vi "OpenDISession.vi"(8 "error in (no error)":errorcluster, 10 "gRPCid":T5, 11 "DIOSessions In":T1={"Array of DI Sessions"=[], "Array of DO Sessions"=[], "Stream ReadDI"={"gRPCid ReadDI"=0, "DISessionName"="", "Stream Status ReadDI"=FALSE, "Async Stop ReadDI Queue"=refnum, "DI Task"="", "ms to wait"=500}}) -> (0 "error out":errorcluster, 3 "DIOSessions Out":T1={"Array of DI Sessions"=[], "Array of DO Sessions"=[], "Stream ReadDI"={"gRPCid ReadDI"=0, "DISessionName"="", "Stream Status ReadDI"=FALSE, "Async Stop ReadDI Queue"=refnum, "DI Task"="", "ms to wait"=500}})   [LabVIEW 2019, in "ctet_dio_User Library.lvlib"]
uses:
  ctet_dio_User Library.lvlib
  Servers/ctet_dio/gRPC lvSupport/Server API/typeDefs/grpcId.ctl
  Types/DIOSessions.ctl
  Types/DISession.ctl
  Types/DOSession.ctl
  Types/StreamReadDI.ctl
  Servers/ctet_dio/ctet_dio Class/RPC Messages/measurementservice_DIOpenSessionResponse/measurementservice_DIOpenSessionResponse_Data.ctl
  Servers/ctet_dio/ctet_dio Class/RPC Messages/measurementservice_ErrorOut/measurementservice_ErrorOut_Data.ctl
  <vilib>/DAQmx/create/channels.llb/DAQmx Create Channel (DI-Digital Input).vi
  Servers/ctet_dio/ctet_dio Class/ctet_dio.lvclass
  Servers/ctet_dio/gRPC lvSupport/gprc-lvsupport.lvlib
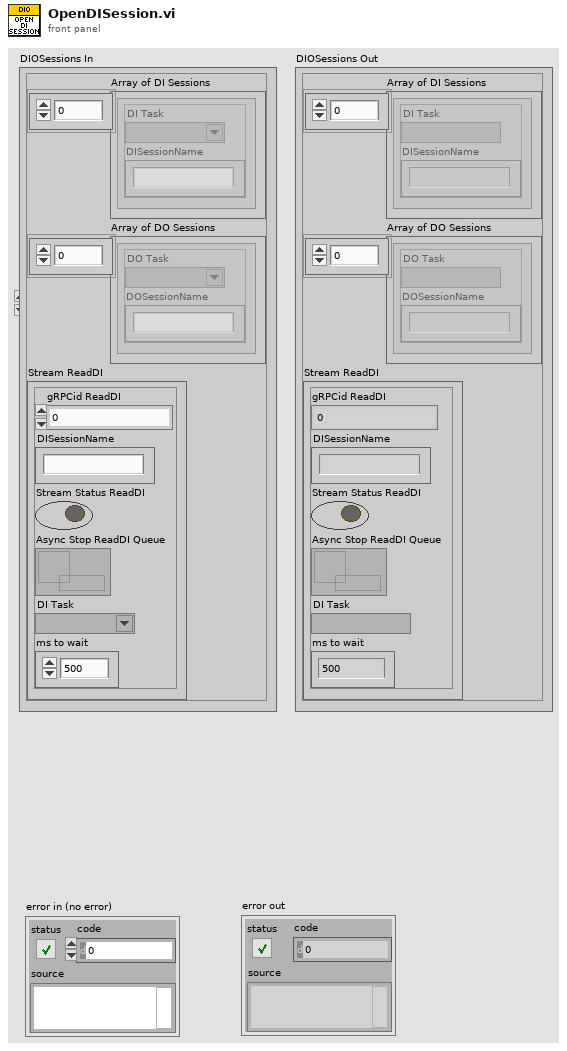
[diagram p1: front panel]
types:
  T1 = typedef "ctet_dio_User Library.lvlib/DIOSessions.ctl" = cluster{"Array of DI Sessions":T2[], "Array of DO Sessions":T3[], "Stream ReadDI":T4}
  T2 = typedef "ctet_dio_User Library.lvlib/DISession.ctl" = cluster{"DI Task":refnum<k21>, "DISessionName":string}
  T3 = typedef "ctet_dio_User Library.lvlib/DOSession.ctl" = cluster{"DO Task":refnum<k21>, "DOSessionName":string}
  T4 = typedef "ctet_dio_User Library.lvlib/StreamReadDI.ctl" = cluster{"gRPCid ReadDI":T5, "DISessionName":string, "Stream Status ReadDI":bool, "Async Stop ReadDI Queue":refnum<queue>, "DI Task":refnum<k21>, "ms to wait":u32}
  T5 = typedef "ctet_dio.lvlib/gprc-lvsupport.lvlib/grpcId.ctl" = u64
  T6 = typedef "ctet_dio.lvlib/ctet_dio.lvclass/measurementservice_ErrorOut_Data.ctl" = cluster{"errCode":i64, "errMessage":string}
  T7 = typedef "ctet_dio.lvlib/ctet_dio.lvclass/measurementservice_DIOpenSessionResponse_Data.ctl" = cluster{"DISessionName":string, "error":T6}
  T8 = typedef "ctet_dio.lvlib/ctet_dio.lvclass/measurementservice_DIOpenSessionRequest_Data.ctl" = cluster{"DISessionName":string, "DIlines":string}
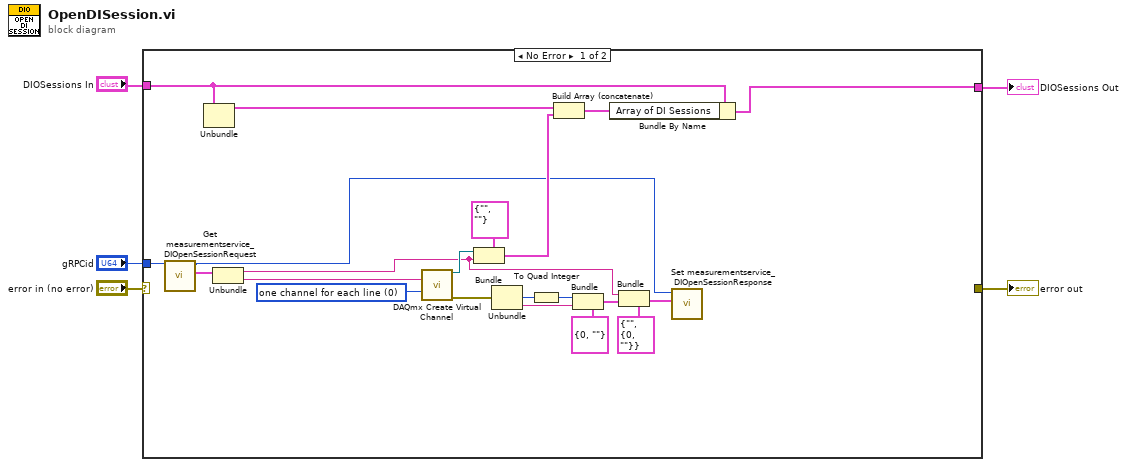
[diagram p0: block diagram]
diagram:
  n1 = case shown="No Error" "error in (no error)" {
    selector: "error in (no error)" -> [_ w28]
    tunnel: [_ w28] -> w5
    tunnel: "gRPCid" -> [w26 _]
    tunnel: "DIOSessions In" -> [w18 w27]
    tunnel: [w17 w27] -> w1
    frame No Error {
      w6 = 0 items=["one channel for each line", "one channel for all lines"] ("line grouping")
      n2 = call "Get measurementservice_DIOpenSessionRequest.vi"("gRPCid"=w26) -> ("Message Data"=w25:T8, "gRPCid out"=w15:T5)  [unwired: 8 in, 1 out]
      n3 = Unbundle(w18) -> ("Array of DI Sessions"=w21:T2[])  [unwired: 2 out]
      n4 = Unbundle(w25) -> ("DISessionName"=w9:string, "DIlines"=w24:string)
      n5 = call-poly <vilib>:"DAQmx Create Virtual Channel.vi"("lines"=w24, "line grouping"=w6) -> ("task out"=w22:refnum<k21>, "error out"=w16:errorcluster)  [unwired: 12 in]
      n6 = Bundle(cluster=T2 {"DI Task"="", "DISessionName"=""} ("DISession"), "DI Task"=w22, "DISessionName"=w9) -> (w20:T2)
      n7 = Unbundle(w16) -> ("code"=w8:i32, "source"=w11:string)  [unwired: 1 out]
      n8 = To Quad Integer(1:w8) -> (0:w7:i64)
      n9 = Build Array (concatenate)(w21, w20) -> (w19:T2[])
      n10 = Bundle(cluster=T6 {"errCode"=0, "errMessage"=""} ("error"), "errCode"=w7, "errMessage"=w11) -> (w10:T6)
      n11 = Bundle By Name(cluster=w18, "Array of DI Sessions"=w19) -> (w17:T1)
      n12 = Bundle(cluster=T7 {"DISessionName"="", "error"={"errCode"=0, "errMessage"=""}} ("measurementservice_DIOpenSessionResponse_Data"), "DISessionName"=w9, "error"=w10) -> (w14:T7)
      n13 = call "Set measurementservice_DIOpenSessionResponse.vi"("Message Data"=w14, "gRPCid"=w15) -> ()  [unwired: 9 in, 1 out]
    }
    frame Error {
    }
  }
  "error out" <- w5
  "DIOSessions Out" <- w1
